vi "Retain last error.vi"(8 "error in (no error)":errorcluster) -> (0 "error out":errorcluster)   [LabVIEW 2020]
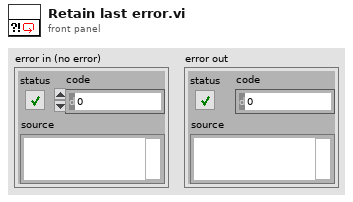
[diagram p1: front panel]
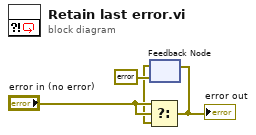
[diagram p0: block diagram]
diagram:
  n1 = feedback #1(errorcluster {"status"=FALSE, "code"=0, "source"=""} ("error in (no error)")) -> (w1:errorcluster)
  n2 = Select(t="error in (no error)", s="error in (no error)", f=w1) -> (s? t:f=w2:errorcluster)
  "error out" <- w2
  n3 = feedback-in #1(w2) -> ()
